vi "Connect.vi"(8 "error in (no error)":errorcluster, 11 "4322 in":refnum<class "4322.lvclass">) -> (0 "error out":errorcluster, 3 "4322 out":refnum<class "4322.lvclass">)   [LabVIEW 2019, in "4322.lvlib" / "4322.lvclass"]
uses:
  Library/4322.lvclass
  C:/Users/Public/Documents/Development/builds/Instruments/Instruments.lvlibp/Library/Instruments.lvclass
  C:/Users/Public/Documents/Development/builds/Instruments/Analog-Output.lvlibp/Library/Analog-Output.lvclass
  Library/4322.lvclass/4322.ctl
  Accessors/Write Local Resource.vi
  builds/Instruments/Instruments.lvlibp/Accessors/Read Resource.vi
  builds/Instruments/Analog-Output.lvlibp/Accessors/Read Channel Names.vi
  <vilib>/DAQmx/create/channels.llb/DAQmx Create Channel (AO-Voltage-Basic).vi
  <resource>/objmgr/daqmx.rc
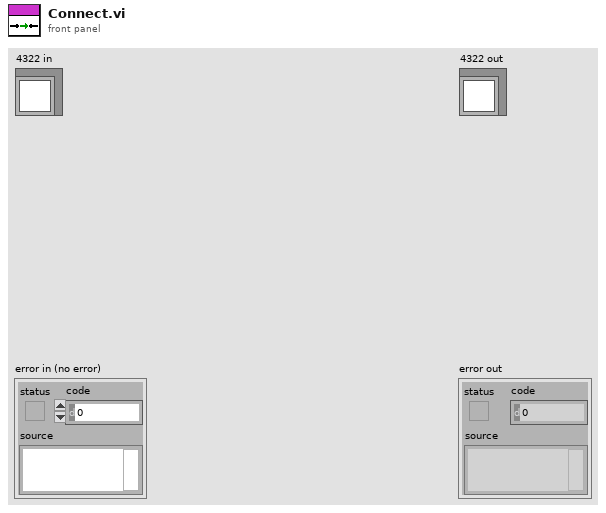
[diagram p1: front panel]
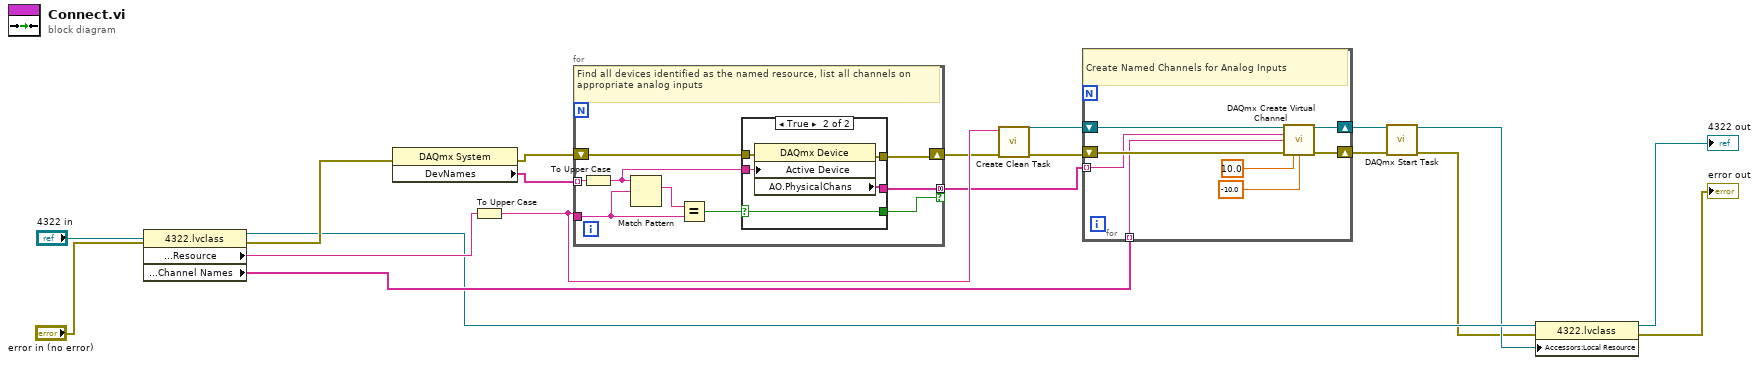
[diagram p0: block diagram]
diagram:
  n1 = property class="4322.lvclass"(reference="4322 in", error in="error in (no error)") -> (reference out=w8:refnum<class "4322.lvclass">, error out=w18:errorcluster, "Accessors:Configuration:Resource"=w16:string, "Accessors:Setting:Channel Names"=w10:string[])
  n2 = property class="DAQmx System"(error in=w18) -> (error out=w17:errorcluster, "DevNames"=w9:tag[])  [unwired: 1 in, 1 out]
  n3 = To Upper Case(1:w16) -> (0:w15:string)
  n4 = for {
    tunnel: w9 -> [w23] mode=indexing
    tunnel: w15 -> [w27]
    shift-right: [w25] -> w14
    shift-left: w17 -> [w24]
    tunnel: [w22] -> w11 mode=concatenating if=w21
    # "Find all devices identified as the named resource, list all channels on appropriate analog inputs"
    n5 = To Upper Case(1:w23) -> (0:w20:string)
    n6 = Match Pattern(string=w20, regular expression=w27) -> (match substring=w28:string)  [unwired: 1 in, 3 out]
    n7 = Equal?(x=w28, y=w27) -> (x = y?=w26:bool)
    n8 = case shown="True" w26 {
      selector: w26 -> [w29 w31]
      tunnel: [w30 w35] -> w25
      tunnel: w24 -> [w30 w34]
      tunnel: w20 -> [_ w33]
      tunnel: [_ w32] -> w22
      tunnel: [w29 w31] -> w21
      frame False {
      }
      frame True {
        n9 = property class="DAQmx Device"(error in=w34, "Active Device"=w33) -> (error out=w35:errorcluster, "AO.PhysicalChans"=w32:tag[])  [unwired: 1 in, 1 out]
      }
    }
  }
  n10 = call "Create Clean Task.vi"("error in (no error)"=w14, "Task Name"=w15) -> ("error out"=w13:errorcluster, "task out"=w12:refnum<k21>)  [unwired: 8 in]
  n11 = for {
    tunnel: w11 -> [w39] mode=indexing
    shift-right: [w43] -> w4
    shift-left: w13 -> [w40]
    shift-right: [w42] -> w3
    shift-left: w12 -> [w41]
    tunnel: w10 -> [w38] mode=indexing
    # "Create Named Channels for Analog Inputs"
    n12 = call-poly <vilib>:"DAQmx Create Virtual Channel.vi"("task in"=w41, "maximum value"=10.0, "minimum value"=-10.0, "physical channels"=w39, "name to assign"=w38, "error in"=w40) -> ("task out"=w42:refnum<k21>, "error out"=w43:errorcluster)  [unwired: 8 in]
  }
  n13 = call <vilib>:"DAQmx Start Task.vi"("task/channels in"=w3, "error in"=w4) -> ("task out"=w2:refnum<k21>, "error out"=w1:errorcluster)  [unwired: 12 in]
  n14 = property class="4322.lvclass"(reference=w8, error in=w1, "Accessors:Local Resource"=w2) -> (reference out=→"4322 out":refnum<class "4322.lvclass">, error out=→"error out":errorcluster)
